vi "Keysight6700 Test.vi"() -> ()   [LabVIEW 2019, in "Wrappers.lvlib"]
uses:
  Wrappers.lvlib
  BSM OOP/Sequence/CodeModules/Hardware Abstraction/Harware Abstraction/Analog out/Analog out.lvclass
panel:
  in  "Setting":T1={"Max. Volt"=10.0, "Current Limit"=0.5, "Volt Level"=10.0}
  in  "6700 Resource":string
  in  "class path":path
  out "Connect?":bool=TRUE
  in  "stop":bool
  out "error out":errorcluster
  out "Measurement":dbl=0.001209082
  in  "Enable Output":bool
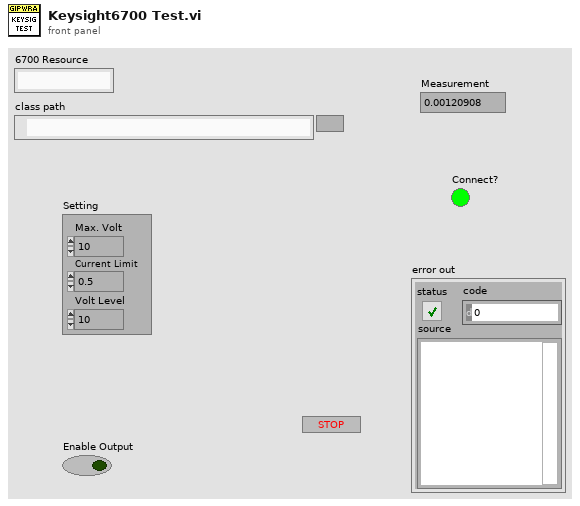
[diagram p1: front panel]
types:
  T1 = cluster{"Max. Volt":dbl, "Current Limit":dbl, "Volt Level":dbl}
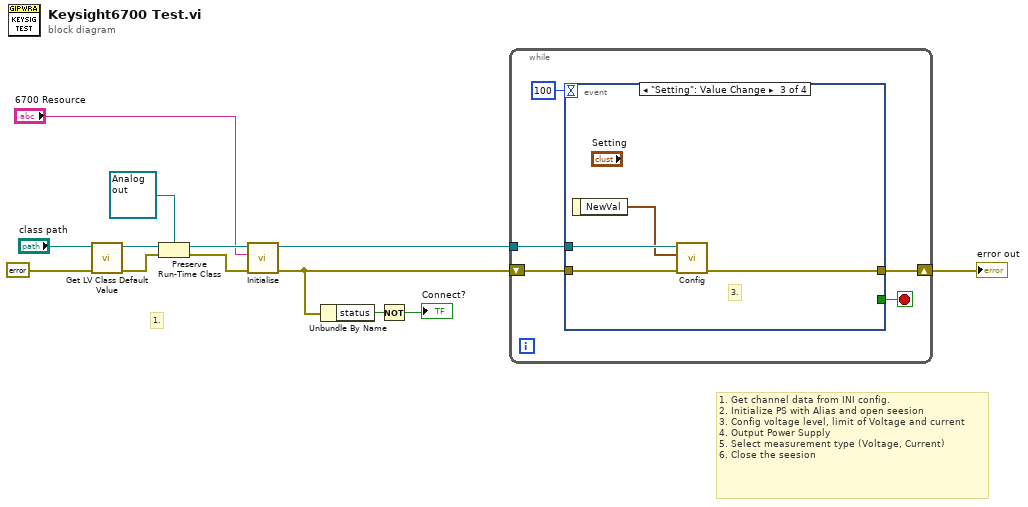
[diagram p0: block diagram]
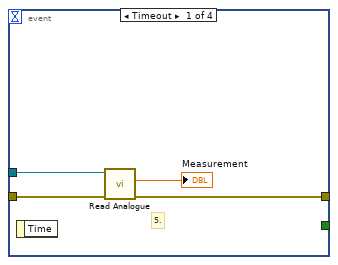
[diagram p2: hidden frame]
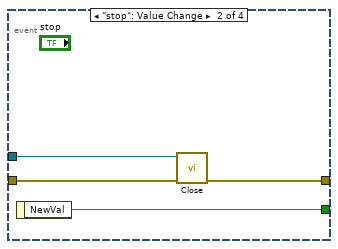
[diagram p3: hidden frame]
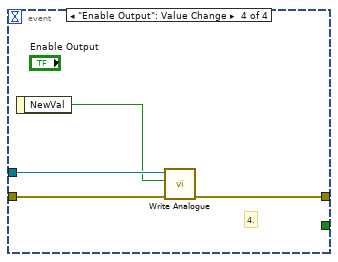
[diagram p4: hidden frame]
diagram:
  # "1. Get channel data from INI config.\n2. Initialize PS with Alias and open seesion \n3. Config voltage level, limit of Voltage and current\n4. Output Power Supply\n5. Select measurement type (Voltage, Current)\n6. Close the seesion"
  # "1."
  n1 = call <vilib>:"Get LV Class Default Value.vi"("error in (no error)"=errorcluster {"status"=FALSE, "code"=0, "source"=""} ("error in"), "class path"="class path") -> ("error out"=w9:errorcluster, "object"=w10:refnum<class>)  [unwired: 8 in]
  n2 = Preserve Run-Time Class(object in=w10, error in=w9, 2:refnum<class "Analog out.lvclass"> refnum ("Hardware Abstration.lvlib:Analog out.lvclass")) -> (object out=w6:refnum<class "Analog out.lvclass">, error out=w5:errorcluster)
  n3 = call-dynamic "Initialise.vi"("error in (no error)"=w5, "Instrument Ref"="6700 Resource", "Instrument in"=w6) -> ("error out"=w2:errorcluster, "Instrument out"=w3:refnum<class "Analog out.lvclass">)  [unwired: 7 in]
  n4 = Unbundle By Name(w2) -> ("status"=w12:bool)
  n5 = Not(x=w12) -> (.not. x?=→"Connect?":bool)
  n6 = while {
    shift-right: [w16] -> w13
    shift-left: w2 -> [w17]
    tunnel: w3 -> [w14]
    stop <- w18 stop-if-true
    n7 = event shown="[2] \"Setting\": Value Change" {
      selector: _ -> [_ _ _ _]
      dyn-events: _ -> [_ _ _ _]
      timeout: 100 -> [_ _ _ _]
      tunnel: [_ w26 _ _] -> w18
      tunnel: [w21 w24 w27 w32] -> w16
      tunnel: w17 -> [w22 w25 w28 w33]
      tunnel: w14 -> [w19 w23 w30 w34]
      event Timeout {
        # "5."
        n8 = event-data() -> ()  [unwired: 1 in, 1 out]
        n9 = call-dynamic "Read Analogue.vi"("error in (no error)"=w22, "Analog out in"=w19) -> ("error out"=w21:errorcluster, "Measurement"=→"Measurement":dbl)  [unwired: 7 in, 1 out]
      }
      event "stop": Value Change {
        n10 = event-data() -> ("NewVal"=w26:bool)  [unwired: 1 in]
        n11 = call-dynamic "Close.vi"("error in (no error)"=w25, "Instrument in"=w23) -> ("error out"=w24:errorcluster)  [unwired: 8 in, 1 out]
      }
      event "Setting": Value Change {
        # "3."
        n12 = event-data() -> ("NewVal"=w29:T1)  [unwired: 1 in]
        n13 = call-dynamic "Config.vi"("error in (no error)"=w28, "Setting"=w29, "Analog out in"=w30) -> ("error out"=w27:errorcluster)  [unwired: 7 in, 1 out]
      }
      event "Enable Output": Value Change {
        # "4."
        n14 = event-data() -> ("NewVal"=w31:bool)  [unwired: 1 in]
        n15 = call-dynamic "Write Analogue.vi"("error in (no error)"=w33, "Outbput"=w31, "PS in"=w34) -> ("error out"=w32:errorcluster)  [unwired: 7 in, 1 out]
      }
    }
  }
  "error out" <- w13
